vi "AUTON_Switch_File.vi"(9 "Number of Auton Files":dbl, 10 "Auton File":dbl=1.0, 11 "Auton Files":string[](array[string])) -> (2 "Current File":string, 3 "Auton Array":dbl[][](array[numeric]))   [LabVIEW 2012]
uses:
  <vilib>/Rock Robotics/WPI/DriverStation/DriverStationLCD/WPI_DriverStationLCDLCDLine.ctl
  <vilib>/Utility/file.llb/Read From Spreadsheet File (DBL).vi
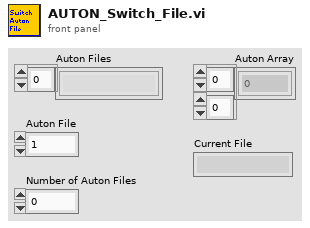
[diagram p1: front panel]
types:
  T1 = typedef "WPI_DriverStationLCDLCDLine.ctl" = enum16{"Main - Line 1", "User - Line 2", "User - Line 3", "User - Line 4", "User - Line 5", "User - Line 6"}
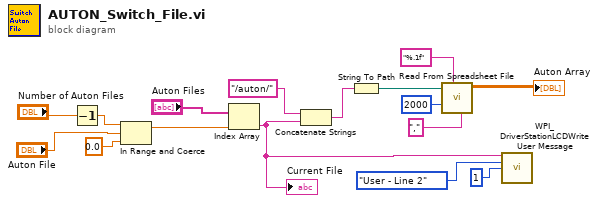
[diagram p0: block diagram]
diagram:
  n1 = Decrement(x="Number of Auton Files") -> (x-1=w3:dbl)
  n2 = In Range and Coerce(upper limit=w3, x="Auton File", lower limit=0.0) -> (coerced(x)=w5:dbl)  [unwired: 1 out]
  n3 = Index Array(array="Auton Files", index=w5) -> (element=w1:string)
  "Current File" <- w1
  n4 = Concatenate Strings("/auton/" ("string"), w1) -> (w13:string)
  n5 = String To Path(string=w13) -> (path=w14:path)
  n6 = call-poly <vilib>:"Read From Spreadsheet File.vi"("delimiter (\\t)"="," ("delimiter (\\t)"), "format (%.3f)"="%.1f", "number of rows (all:-1)"=2000, "file path (dialog if empty)"=w14) -> ("all rows"=→"Auton Array":dbl[][])  [unwired: 1 in, 6 out]
  n7 = call <vilib>:"WPI_DriverStationLCDWrite User Message.vi"("line text"=w1, "line"=WPI_DriverStationLCDLCDLine."User - Line 2", "starting column"=i8 1) -> ()  [unwired: 2 in, 11 out]
